vi "instrument helloworld.vi"() -> ()   [LabVIEW 2016]
panel:
  out "error out":errorcluster
  out "IDN Response":string
  in  "VISA resource name":refnum<visa-resource-name>
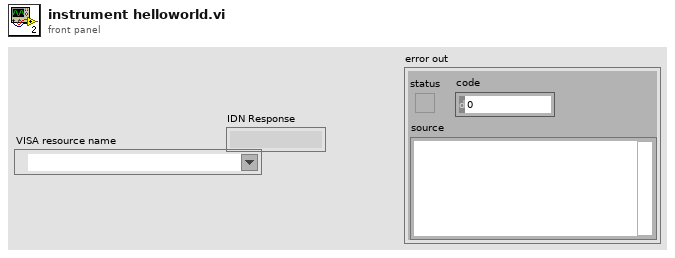
[diagram p1: front panel]
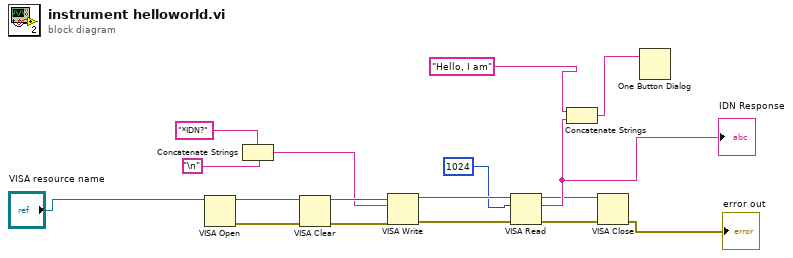
[diagram p0: block diagram]
diagram:
  n1 = VISA Open(VISA resource name="VISA resource name") -> (VISA resource name=w16:refnum<visa-resource-name>, error out=w13:errorcluster)  [unwired: 4 in]
  n2 = Concatenate Strings("*IDN?", "\n") -> (w8:string)
  n3 = VISA Clear(VISA resource name=w16, error in (no error)=w13) -> (VISA resource name out=w15:refnum<visa-resource-name>, error out=w12:errorcluster)
  n4 = VISA Write(VISA resource name=w15, write buffer=w8, error in (no error)=w12) -> (VISA resource name out=w14:refnum<visa-resource-name>, error out=w11:errorcluster)  [unwired: 1 out]
  n5 = VISA Read(VISA resource name=w14, byte count=1024, error in (no error)=w11) -> (VISA resource name out=w3:refnum<visa-resource-name>, read buffer=w4:string, error out=w2:errorcluster)  [unwired: 1 out]
  "IDN Response" <- w4
  n6 = Concatenate Strings("Hello, I am", w4) -> (w5:string)
  n7 = VISA Close(VISA resource name=w3, error in (no error)=w2) -> (error out=→"error out":errorcluster)
  n8 = One Button Dialog(message=w5) -> ()  [unwired: 1 in, 1 out]
